vi "Turn.vi"(0 "reinitialize?":bool, 4 "Delta?":bool, 6 "Start Turn":bool=TRUE, 7 "output range":cluster{"output high":dbl, "output low":dbl}={"output high"=1.0, "output low"=-1.0}, 8 "Negate":bool, 9 "PID gains":T1={"proportional gain (Kc)"=1.0, "integral time (Ti, min)"=0.01, "derivative time (Td, min)"=0.0} {"derivative time (Td, min)" format="%.3f"; "integral time (Ti, min)" format="%.3f"; "proportional gain (Kc)" format="%.3f"}, 10 "Desired Angle":dbl, 11 "Current Angle":dbl) -> (1 "Delta Angle Remaining":dbl, 2 "Setpoint":dbl, 3 "Cheesy Steer":dbl, 5 "Turn Hold Point":dbl)   [LabVIEW 2015]
uses:
  <vilib>/addons/control/pid/pid.llb/PID (DBL).vi
  <vilib>/addons/control/pid/NI_PID_pid.lvlib
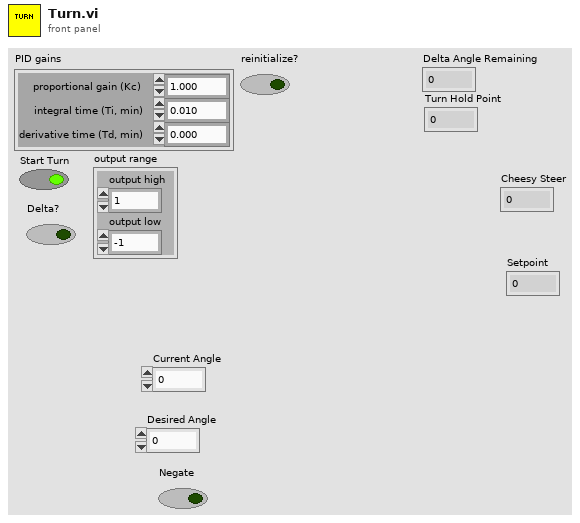
[diagram p1: front panel]
types:
  T1 = cluster{"proportional gain (Kc)":dbl, "integral time (Ti, min)":dbl, "derivative time (Td, min)":dbl}
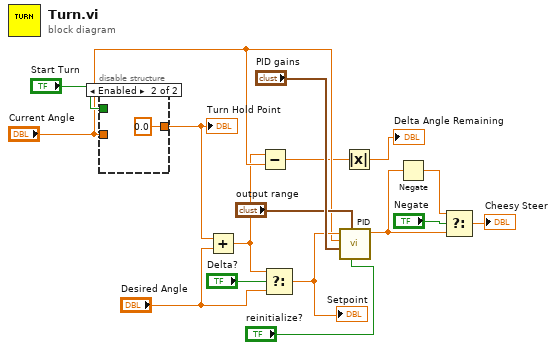
[diagram p0: block diagram]
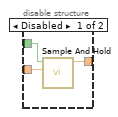
[diagram p2: hidden frame]
diagram:
  n1 = disable-structure shown="Enabled" {
    disable-tunnel: "Start Turn" -> [w19 _]
    disable-tunnel: [w18 0.0 ("Turn Hold Point")] -> w14
    disable-tunnel: "Current Angle" -> [w17 _]
    frame Disabled {
      n2 = call "Sample And Hold.vi"("Signal"=w17, "Condition"=w19) -> ("Signal Out"=w18:dbl)  [unwired: 9 in]
    }
    frame Enabled {
    }
  }
  "Turn Hold Point" <- w14
  n3 = Add(x=w14, y="Desired Angle") -> (x+y=w2:dbl)
  n4 = Subtract(x=w2, y="Current Angle") -> (x-y=w5:dbl)
  n5 = Select(t=w2, s="Delta?", f="Desired Angle") -> (s? t:f=w8:dbl)
  "Setpoint" <- w8
  n6 = call-poly <vilib>:"PID.vi"("reinitialize? (F)"="reinitialize?", "output range"="output range", "PID gains"="PID gains", "process variable"="Current Angle", "setpoint"=w8) -> ("output"=w12:dbl)  [unwired: 5 in, 1 out]
  n7 = Absolute Value(x=w5) -> (abs(x)=→"Delta Angle Remaining":dbl)
  n8 = Negate(x=w12) -> (-x=w11:dbl)
  n9 = Select(t=w11, s="Negate", f=w12) -> (s? t:f=→"Cheesy Steer":dbl)
